vi "SubVI_ReadMatB_001.vi"(10 "# Bands":i32, 11 "1-bit pixmap   in":bool[][](array[boolean])) -> (2 "array of inputs":i32[](array[numeric]), 3 "total #iter":i32)   [LabVIEW 2018]
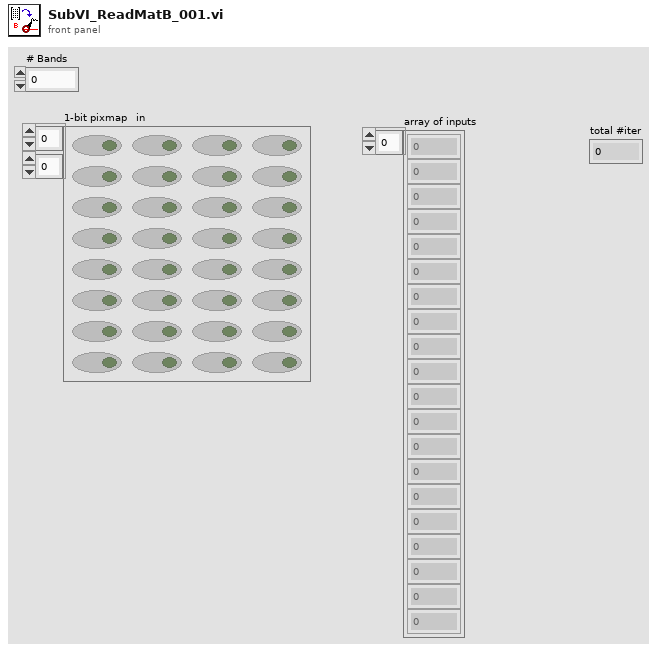
[diagram p1: front panel]
types:
  T1 = cluster{"[0]":i32, "[1]":i32, "[2]":i32, "[3]":i32, "[4]":i32, "[5]":i32, "[6]":i32, "[7]":i32, "[8]":i32}
  T2 = cluster{"[0]":dbl, "[1]":dbl, "[2]":dbl, "[3]":dbl, "[4]":dbl, "[5]":dbl, "[6]":dbl, "[7]":dbl, "[8]":dbl}
  T3 = cluster{"[0]":i32, "[1]":i32, "[0]":i32, "[1]":i32}
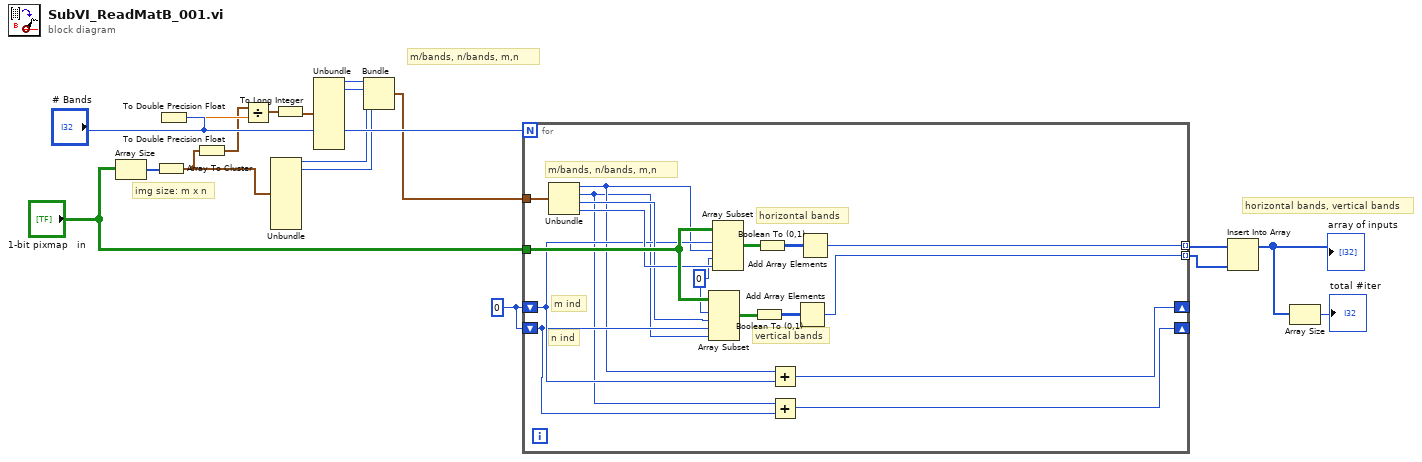
[diagram p0: block diagram]
diagram:
  w5 = 0
  # "img size: m x n"
  # "horizontal bands, vertical bands"
  # "m/bands, n/bands, m,n"
  n1 = Array Size(array="1-bit pixmap   in") -> (size(s)=w18:i32[])
  n2 = Array To Cluster(array=w18) -> (cluster=w13:T1)
  n3 = To Double Precision Float(number="# Bands") -> (double precision float=w15:dbl)
  n4 = To Double Precision Float(number=w13) -> (double precision float=w14:T2)
  n5 = Divide(x=w14, y=w15) -> (x/y=w12:T2)
  n6 = Unbundle(w13) -> ("[0]"=w8:i32, "[1]"=w7:i32)  [unwired: 7 out]
  n7 = To Long Integer(number=w12) -> (32bit integer=w11:T1)
  n8 = Unbundle(w11) -> ("[0]"=w10:i32, "[1]"=w9:i32)  [unwired: 7 out]
  n9 = Bundle("[0]"=w10, "[1]"=w9, "[0]"=w8, "[1]"=w7) -> (w6:T3)  [unwired: 1 in]
  n10 = for {
    N: "# Bands" -> [_]
    shift-right: [w26] -> _
    shift-left: w5 -> [w30]
    tunnel: "1-bit pixmap   in" -> [w34]
    tunnel: w6 -> [w35]
    shift-right: [w25] -> _
    shift-left: w5 -> [w29]
    tunnel: [w20] -> w4 mode=indexing
    tunnel: [w19] -> w3 mode=indexing
    w31 = 0
    # "horizontal bands"
    # "vertical bands"
    # "n ind"
    # "m ind"
    # "m/bands, n/bands, m,n"
    n11 = Unbundle(w35) -> ("[0]"=w28:i32, "[1]"=w27:i32, "[0]"=w32:i32, "[1]"=w33:i32)
    n12 = Array Subset(array=w34, index (row)=w31, length (row)=w32, index (col)=w29, length (col)=w27) -> (w21:bool[][])
    n13 = Array Subset(array=w34, index (row)=w30, length (row)=w28, index (col)=w31, length (col)=w33) -> (w24:bool[][])
    n14 = Boolean To (0,1)(Boolean=w21) -> (0, 1=w22:i16[][])
    n15 = Boolean To (0,1)(Boolean=w24) -> (0, 1=w23:i16[][])
    n16 = Add(x=w28, y=w30) -> (x+y=w26:i32)
    n17 = Add(x=w27, y=w29) -> (x+y=w25:i32)
    n18 = Add Array Elements(numeric array=w22) -> (sum=w19:i16)
    n19 = Add Array Elements(numeric array=w23) -> (sum=w20:i16)
  }
  n20 = Insert Into Array(array=w4, new element=w3) -> (w2:i16[])  [unwired: 1 in]
  "array of inputs" <- w2
  n21 = Array Size(array=w2) -> (size(s)=→"total #iter":i32)
